vi "LoadNewGame.vi"(8 "error in (no error)":errorcluster, 10 "NewGame":refnum<class "Game.lvclass">, 11 "Game in":refnum<class "Game.lvclass">) -> (0 "error out":errorcluster, 3 "Game out":refnum<class "Game.lvclass">)   [LabVIEW 2019, in "RT_Game.lvlib" / "Game.lvclass"]
uses:
  Game.lvclass
  Game.lvclass/Game.ctl
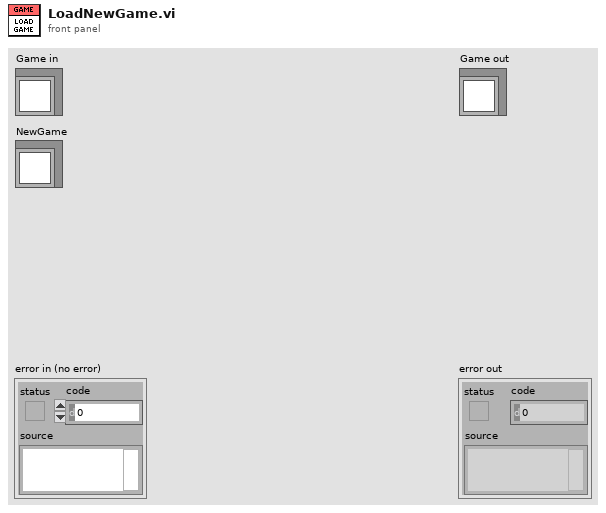
[diagram p1: front panel]
types:
  T1 = typedef "FPGA_Interface.ctl" = refnum<k20>
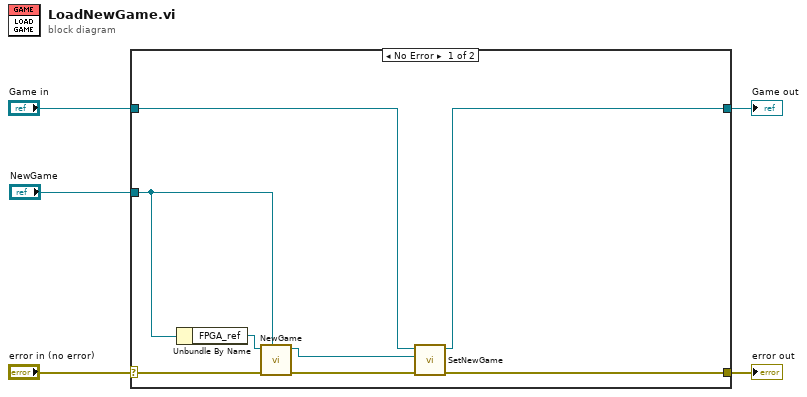
[diagram p0: block diagram]
diagram:
  n1 = case shown="No Error" "error in (no error)" {
    selector: "error in (no error)" -> [w13 w15]
    tunnel: [w12 w15] -> w4
    tunnel: [w10 w14] -> w2
    tunnel: "Game in" -> [w11 w14]
    tunnel: "NewGame" -> [w6 _]
    frame No Error {
      n2 = Unbundle By Name(w6) -> ("FPGA_ref"=w7:T1)
      n3 = call-dynamic "NewGame.vi"("GameType (ChildObject)"=w6, "error in (no error)"=w13, "FPGA_ref"=w7) -> ("error out"=w9:errorcluster, "Game out"=w8:refnum<class "Game.lvclass">)  [unwired: 7 in]
      n4 = call "SetNewGame.vi"("error in (no error)"=w9, "NewGame"=w8, "Game in"=w11) -> ("error out"=w12:errorcluster, "Game out"=w10:refnum<class "Game.lvclass">)  [unwired: 7 in]
    }
    frame Error {
    }
  }
  "error out" <- w4
  "Game out" <- w2
